vi "Separate ROI.vi"(4 "Axis":bool, 6 "SearchArea":dbl=0.5 format="%#_13g", 7 "ROI Descriptor":T1 {"Contours"."Type" items=["No Selection", "Point", "Line", "Rectangle", "Oval", "Polygon", "Freehand Region", "Annulus", "Unused2", "Unused3", "Broken Line", "Freehand Line", "Rotated Rectangle"]}) -> (2 "Right/Bottom ROI":T2 {"Contours"."Type" items=["No Selection", "Point", "Line", "Rectangle", "Oval", "Polygon", "Free", "Annulus", "Unused2", "Unused3", "Broken Line", "Free Hand Line", "Rotated Rectangle"]}, 3 "Left/Top ROI":T2 {"Contours"."Type" items=["No Selection", "Point", "Line", "Rectangle", "Oval", "Polygon", "Free", "Annulus", "Unused2", "Unused3", "Broken Line", "Free Hand Line", "Rotated Rectangle"]})   [LabVIEW 2015]
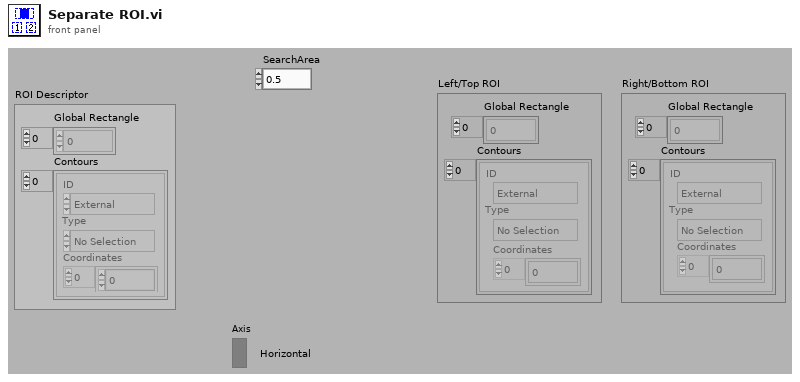
[diagram p1: front panel]
types:
  T1 = typedef "ROI Descriptor" = cluster{"Global Rectangle":i32[], "Contours":cluster{"ID":enum32{"External", "Internal"}, "Type":u32, "Coordinates":i32[]}[]}
  T2 = cluster{"Global Rectangle":i32[], "Contours":cluster{"ID":enum32{"External", "Internal"}, "Type":u32, "Coordinates":i32[]}[]}
  T3 = cluster{"ID":enum32{"External", "Internal"}, "Type":u32, "Coordinates":i32[]}[]
  T4 = cluster{"ID":enum32{"External", "Internal"}, "Type":u32, "Coordinates":i32[]}
  T5 = enum32{"No Selection", "Point", "Line", "Rectangle", "Oval", "Polygon", "Free", "Unused1", "Unused2", "Unused3", "Broken Line", "Free Hand Line"}
  T6 = cluster{"ID":enum32{"External", "Internal"}, "Type":enum32{"No Selection", "Point", "Line", "Rectangle", "Oval", "Polygon", "Free", "Unused1", "Unused2", "Unused3", "Broken Line", "Free Hand Line"}, dbl[]}
  T7 = cluster{"ID":enum32{"External", "Internal"}, "Type":enum32{"No Selection", "Point", "Line", "Rectangle", "Oval", "Polygon", "Free", "Unused1", "Unused2", "Unused3", "Broken Line", "Free Hand Line"}, dbl[]}[]
  T8 = cluster{"Global Rectangle":i32[], cluster{"ID":enum32{"External", "Internal"}, "Type":enum32{"No Selection", "Point", "Line", "Rectangle", "Oval", "Polygon", "Free", "Unused1", "Unused2", "Unused3", "Broken Line", "Free Hand Line"}, dbl[]}[]}
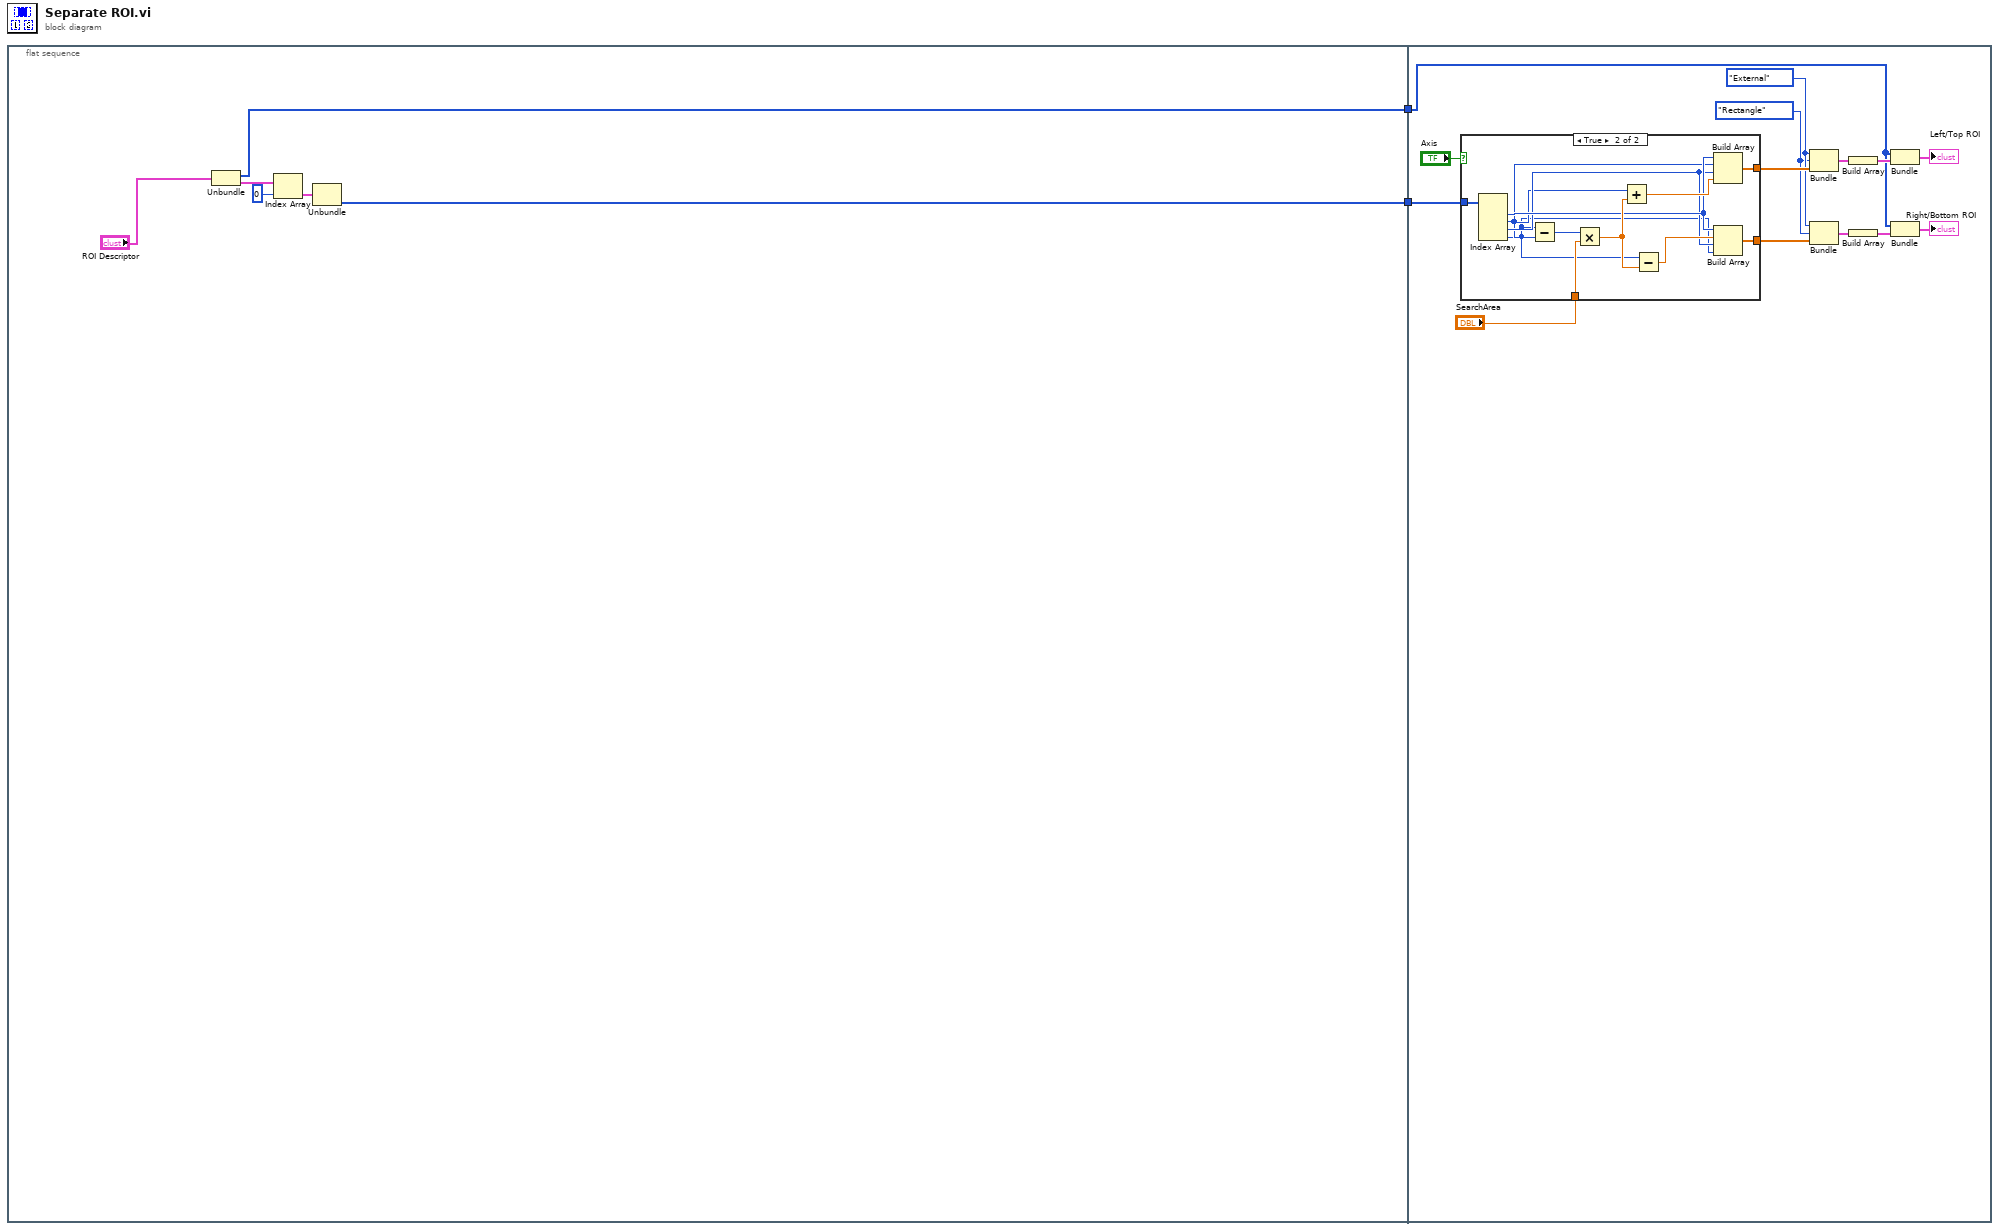
[diagram p0: block diagram]
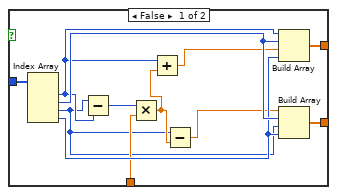
[diagram p2: hidden frame]
diagram:
  n1 = flat-sequence {
    tunnel: [w5] -> w2
    tunnel: [w4] -> w1
    tunnel: w2 -> [w20]
    tunnel: w1 -> [w19]
    frame #0 {
      n2 = Unbundle("ROI Descriptor") -> ("Global Rectangle"=w5:i32[], "Contours"=w6:T3)
      n3 = Index Array(array=w6, index=0 ("Index")) -> (element=w8:T4)
      n4 = Unbundle(w8) -> ("Coordinates"=w4:i32[])  [unwired: 2 out]
    }
    frame #1 {
      w11 = T5."Rectangle" ("Type")
      w12 = enum32{"External", "Internal"}."External" ("ID")
      n5 = case shown="True" "Axis" {
        tunnel: w19 -> [w33 w45]
        tunnel: [w30 w44] -> w18
        tunnel: [w29 w43] -> w17
        tunnel: "SearchArea" -> [w28 w42]
        frame False {
          n6 = Index Array(array=w33) -> (element #1=w24:i32, element #2=w32:i32, element #3=w23:i32, element #4=w31:i32)  [unwired: 4 in]
          n7 = Subtract(x=w23, y=w24) -> (x-y=w34:i32)
          n8 = Multiply(x=w34, y=w28) -> (x*y=w27:dbl)
          n9 = Add(x=w24, y=w27) -> (x+y=w26:dbl)
          n10 = Subtract(x=w23, y=w27) -> (x-y=w25:dbl)
          n11 = Build Array(w24, w32, w26, w31) -> (w30:dbl[])
          n12 = Build Array(w25, w32, w23, w31) -> (w29:dbl[])
        }
        frame True {
          n13 = Index Array(array=w45) -> (element #1=w38:i32, element #2=w36:i32, element #3=w37:i32, element #4=w35:i32)  [unwired: 4 in]
          n14 = Subtract(x=w35, y=w36) -> (x-y=w46:i32)
          n15 = Multiply(x=w46, y=w42) -> (x*y=w41:dbl)
          n16 = Add(x=w36, y=w41) -> (x+y=w39:dbl)
          n17 = Subtract(x=w35, y=w41) -> (x-y=w40:dbl)
          n18 = Build Array(w38, w36, w37, w39) -> (w44:dbl[])
          n19 = Build Array(w38, w40, w37, w35) -> (w43:dbl[])
        }
      }
      n20 = Bundle("ID"=w12, "Type"=w11, w18) -> (w16:T6)  [unwired: 1 out]
      n21 = Bundle("ID"=w12, "Type"=w11, w17) -> (w15:T6)  [unwired: 1 out]
      n22 = Build Array(w16) -> (w22:T7)
      n23 = Build Array(w15) -> (w21:T7)
      n24 = Bundle("Global Rectangle"=w20, w22) -> (→"Left/Top ROI":T8)  [unwired: 1 out]
      n25 = Bundle("Global Rectangle"=w20, w21) -> (→"Right/Bottom ROI":T8)  [unwired: 1 out]
    }
  }
